vi "Get SDF Path from INI.vi"(8 "error in (no error)":errorcluster, 11 "INI File Path":path) -> (0 "error out":errorcluster, 3 "SDF File Path":path, 4 "Valid Path?":bool)   [LabVIEW 2016, in "System Mapping Tool.lvlib"]
uses:
  System Mapping Tool.lvlib
  <vilib>/Utility/config.llb/NI_LVConfig.lvlib
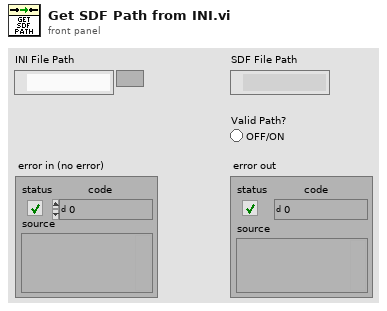
[diagram p1: front panel]
types:
  T1 = typedef "NI_LVConfig.lvlib/Config Data RefNum.ctl" = refnum<k1>
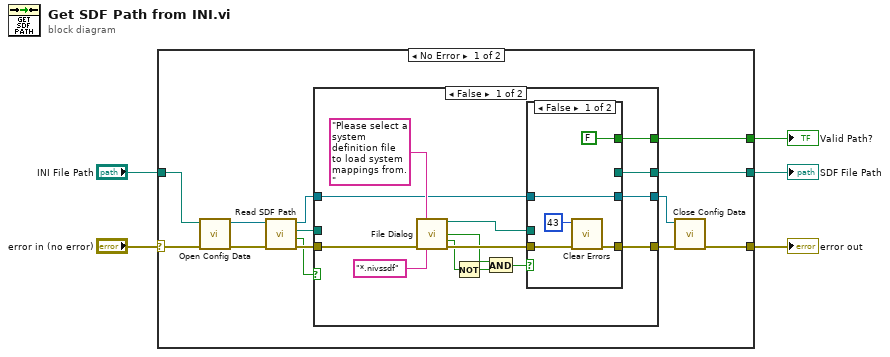
[diagram p0: block diagram]
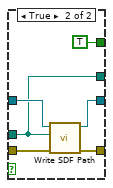
[diagram p2: hidden frame]
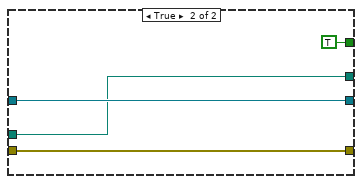
[diagram p3: hidden frame]
diagram:
  n1 = case shown="No Error" "error in (no error)" {
    selector: "error in (no error)" -> [w18 w48]
    tunnel: [w10 w48] -> w4
    tunnel: "INI File Path" -> [w17 _]
    tunnel: [w7 _] -> w2
    tunnel: [w6 _] -> w1
    frame No Error {
      n2 = call <vilib>:"Open Config Data.vi"("error in (no error)"=w18, "configuration file path"=w17) -> ("error out"=w16:errorcluster, "refnum"=w15:T1)  [unwired: 7 in, 1 out]
      n3 = call "Read SDF Path.vi"("error in (no error)"=w16, "refnum"=w15) -> ("error out"=w14:errorcluster, "Found?"=w13:bool, "Path"=w11:path, "refnum out"=w12:T1)  [unwired: 6 in]
      n4 = case shown="False" w13 {
        tunnel: w14 -> [w30 w47]
        tunnel: w12 -> [w22 w46]
        tunnel: w11 -> [_ w45]
        tunnel: [w28 w47] -> w9
        tunnel: [w21 w46] -> w8
        tunnel: [w20 w45] -> w7
        tunnel: [w19 TRUE] -> w6
        frame False {
          n5 = call "File Dialog"("prompt"="Please select a system definition file to load system mappings from.", "error in"=w30, "pattern (all files)"="*.nivssdf") -> ("selected path"=w27:path, "exists"=w26:bool, "cancelled"=w24:bool, "error out"=w29:errorcluster)  [unwired: 9 in]
          n6 = Not(x=w24) -> (.not. x?=w25:bool)
          n7 = And(x=w26, y=w25) -> (x .and. y?=w23:bool)
          n8 = case shown="False" w23 {
            tunnel: w29 -> [w36 w43]
            tunnel: [w34 w42] -> w28
            tunnel: w27 -> [_ w39]
            tunnel: w22 -> [w37 w41]
            tunnel: [w37 w40] -> w21
            tunnel: [_ w39] -> w20
            tunnel: [FALSE TRUE] -> w19
            frame False {
              n9 = call <vilib>:"Clear Errors.vi"("error in (no error)"=w36, "specific error code to clear (0: all)"=43) -> ("error out"=w34:errorcluster)  [unwired: 4 in, 1 out]
            }
            frame True {
              n10 = call "Write SDF Path.vi"("error in (no error)"=w43, "Path"=w39, "refnum"=w41) -> ("error out"=w42:errorcluster, "refnum out"=w40:T1)  [unwired: 7 in]
            }
          }
        }
        frame True {
        }
      }
      n11 = call <vilib>:"Close Config Data.vi"("error in (no error)"=w9, "refnum"=w8) -> ("error out"=w10:errorcluster)  [unwired: 8 in, 1 out]
    }
    frame Error {
    }
  }
  "SDF File Path" <- w2
  "error out" <- w4
  "Valid Path?" <- w1
